vi "DataTypesExample.vi"() -> ()   [LabVIEW 2020]
uses:
  <vilib>/measure/NI_MABase.lvlib
panel:
  in  "Tab":T1(tab)
  in  "Liczba 1":dbl=15.1
  in  "Liczba 3":dbl=3.0
  in  "Liczba 2":i32=20
  out "Wynik 2":u16
  out "Wynik 1":dbl
  in  "Liczba 4":dbl=2.0
  in  "Tak/nie":bool
  in  "Prawda/falsz 2":bool
  in  "Prawda/falsz":bool
  out "Wynik logiczny":bool
  out "Tak/nie liczbowo":i16
  in  "Combo Box":string(combo)=" tekst 1"
  in  "Sciezka":path=path "D:/LabVIEW Workspace/Kanał na YT/Główne repozytorium kanału/LabVIEW Tutorial #2/DataTypesExample.vi"
  in  "Teskt 2":string="KOTA"
  in  "Teskt 1":string="ALA MA"
  out "Tekst polaczony":string
  out "Liczba na tekst":string
  in  "Liczba":i32=5
  out "Sciezka tekstowo":string
  out "Tekst z combo boxa":string
  out "error out":errorcluster
  in  "error in (no error)":errorcluster
  in  "Liczba do klastra 1":dbl=367.0
  out "Cluster":cluster{"Liczba 1 ":dbl, "Liczba 2":dbl}
  in  "Klaster 1":T2={"Liczba"=22.0, "Prawda fałsz"=TRUE, "Tekst"="TO Z KLASTRA"}
  out "Liczba 6":dbl
  in  "Liczba do klastra 2":dbl=211.22
  out "Prawda fałsz":bool
  out "Tekst":string
  in  "Tablica klastrów":cluster{"PRAWDA/FAŁSZ":bool, "Tekst":string}[](array[cluster])=[{"PRAWDA/FAŁSZ"=TRUE, "Tekst"="test1"}, {"PRAWDA/FAŁSZ"=FALSE, "Tekst"="test2"}, {"PRAWDA/FAŁSZ"=TRUE, "Tekst"="test3"}]
  in  "Tablica tekst":string[](array[string])=["1", "2", "3"]
  in  "TABLICA  2D":dbl[][](array[numeric])=[[1.0, 2.0, 3.0], [4.0, 5.0, 6.0]]
  in  "TABLICA":dbl[](array[numeric])=[1.0, 2.0, 3.0, 4.0]
  out "Wybrany element 1":dbl
  out "Wybrany element 2":dbl
  in  "VISA resource name":refnum<visa-resource-name>
  out "Graf":waveform(dbl)(graph)={"t0"=timestamp(0 s since 1904-01-01), "dt"=0.001, "Y"=array[1000 elements]}
  in  "Ctl Refnum":refnum<vi>
  out "LabVIEW Object Out":refnum<class>
  in  "LabVIEW Object In":refnum<class>
  out "Ctl Refnum 2":refnum<vi>
  out "signal out":waveform(dbl)={"t0"=timestamp(0 s since 1904-01-01), "dt"=0.001, "Y"=array[1000 elements]}
  out "Variant":variant=variant(dbl 10.0)
  out "Liczba z warianta":dbl=10.0
  # "Klikamy prawym -> Paleta Numeric"
  # "Klikamy prawym -> Paleta Boolean"
  # "Klikamy prawym -> Paleta String&Paths"
  # "Klikamy prawym -> Paleta Data Containers"
  # "Klikamy prawym -> Paleta Data Containers"
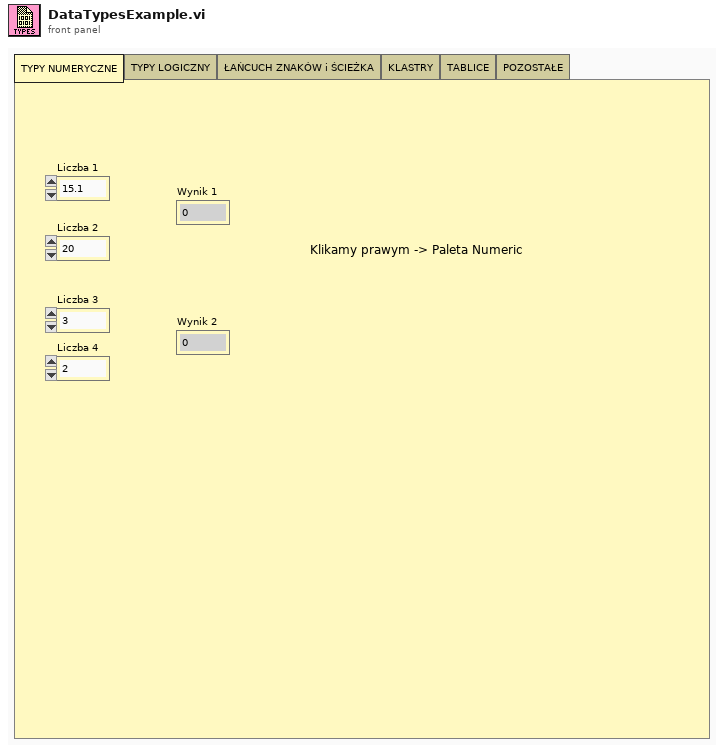
[diagram p1: front panel]
types:
  T1 = enum32{"TYPY NUMERYCZNE", "TYPY LOGICZNY", "ŁAŃCUCH ZNAKÓW i ŚCIEŻKA", "KLASTRY", "TABLICE", "POZOSTAŁE"}
  T2 = cluster{"Liczba":dbl, "Prawda fałsz":bool, "Tekst":string}
  T3 = cluster{"Liczba do klastra 1 ":dbl, "Liczba do klastra 2":dbl}
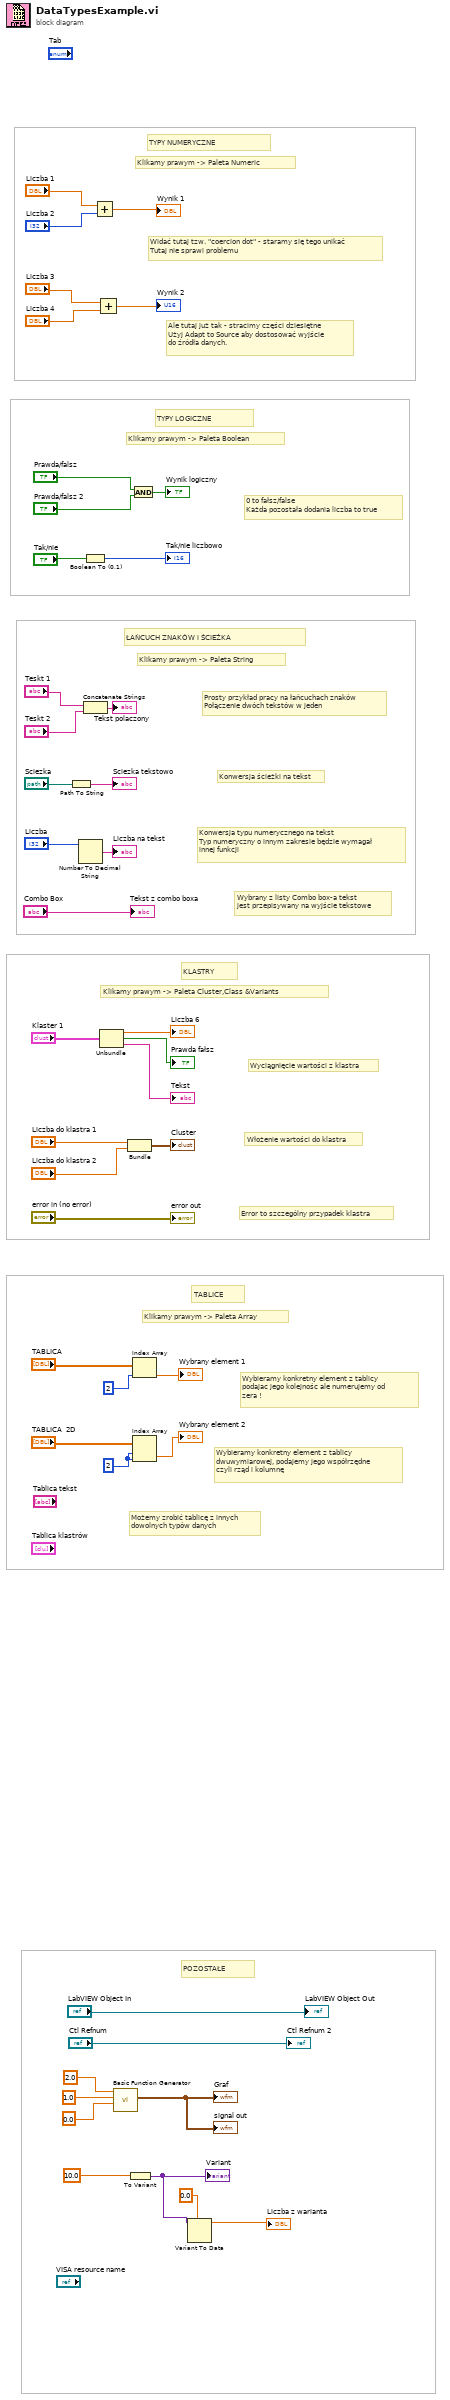
[diagram p0: block diagram]
diagram:
  w16 = 2 ("index")
  # "Ale tutaj już tak - stracimy części dziesiętne\nUżyj Adapt to Source aby dostosować wyjście\ndo źródła danych."
  # "Wybieramy konkretny element z tablicy\ndwuwymiarowej, podajemy jego współrzędne\nczyli rząd i kolumnę"
  # "Wybieramy konkretny element z tablicy\npodajac jego kolejnośc ale numerujemy od\nzera !"
  # "Konwersja ścieżki na tekst"
  # "Prosty przykład pracy na łańcuchach znaków\nPołączenie dwóch tekstów w jeden"
  # "Wybrany z listy Combo box-a tekst\njest przepisywany na wyjście tekstowe"
  # "Konwersja typu numerycznego na tekst\nTyp numeryczny o innym zakresie będzie wymagał\ninnej funkcji"
  # "Klikamy prawym -> Paleta Array"
  # "Klikamy prawym -> Paleta Cluster,Class &Variants"
  # "Klikamy prawym -> Paleta String"
  # "Klikamy prawym -> Paleta Boolean"
  # "Klikamy prawym -> Paleta Numeric"
  # "Error to szczególny przypadek klastra"
  # "Włożenie wartości do klastra"
  # "Możemy zrobić tablicę z innych\ndowolnych typów danych"
  # "Wyciągnięcie wartości z klastra"
  # "0 to fałsz/false\nKażda pozostała dodania liczba to true"
  # "POZOSTAŁE"
  # "TABLICE"
  # "KLASTRY"
  # "ŁAŃCUCH ZNAKÓW i ŚCIEŻKA"
  # "TYPY LOGICZNE"
  # "TYPY NUMERYCZNE"
  # "Widać tutaj tzw. \"coercion dot\" - staramy się tego unikać\nTutaj nie sprawi problemu"
  n1 = Path To String(path="Sciezka") -> (string=→"Sciezka tekstowo":string)
  n2 = Number To Decimal String(number="Liczba") -> (decimal integer string=→"Liczba na tekst":string)  [unwired: 1 in]
  n3 = Boolean To (0,1)(Boolean="Tak/nie") -> (0, 1=→"Tak/nie liczbowo":i16)
  n4 = Concatenate Strings("Teskt 1", "Teskt 2") -> (→"Tekst polaczony":string)
  n5 = Add(x="Liczba 1", y="Liczba 2") -> (x+y=→"Wynik 1":dbl)
  n6 = Add(x="Liczba 3", y="Liczba 4") -> (x+y=→"Wynik 2":dbl)
  n7 = Unbundle("Klaster 1") -> ("Liczba"=→"Liczba 6":dbl, "Prawda fałsz"=→"Prawda fałsz":bool, "Tekst"=→"Tekst":string)
  n8 = call <vilib>:"Basic Function Generator.vi"("phase"=0.0, "amplitude"=1.0, "frequency"=2.0) -> ("signal out"=→"Graf" →"signal out":waveform(dbl))  [unwired: 6 in, 2 out]
  n9 = Bundle("Liczba do klastra 1"="Liczba do klastra 1", "Liczba do klastra 2"="Liczba do klastra 2") -> (→"Cluster":T3)  [unwired: 1 in]
  n10 = To Variant(anything=10.0 ("phase")) -> (Variant=w7:variant)
  "Variant" <- w7
  n11 = And(x="Prawda/falsz", y="Prawda/falsz 2") -> (x .and. y?=→"Wynik logiczny":bool)
  n12 = Index Array(array="TABLICA", index=2) -> (element=→"Wybrany element 1":dbl)
  n13 = Index Array(array="TABLICA  2D", index (row)=w16, index (col)=w16) -> (element=→"Wybrany element 2":dbl)
  n14 = Variant To Data(type=0.0 ("phase"), Variant=w7) -> (data=→"Liczba z warianta":dbl)  [unwired: 1 in, 1 out]
  "error out" <- "error in (no error)"
  "LabVIEW Object Out" <- "LabVIEW Object In"
  "Ctl Refnum 2" <- "Ctl Refnum"
  "Tekst z combo boxa" <- "Combo Box"
